vi "hamilton_controller_shunt2.vi"(8 "error in":errorcluster, 9 "Open?":bool, 10 "valve":enum16{"A", "B", "C", "D", "ALL", "E"}(ring), 11 "action":T1(ring)) -> (0 "error out":errorcluster)   [LabVIEW 2013]
uses:
  <vilib>/Instr/_visa.llb/VISA Configure Serial Port (Instr).vi
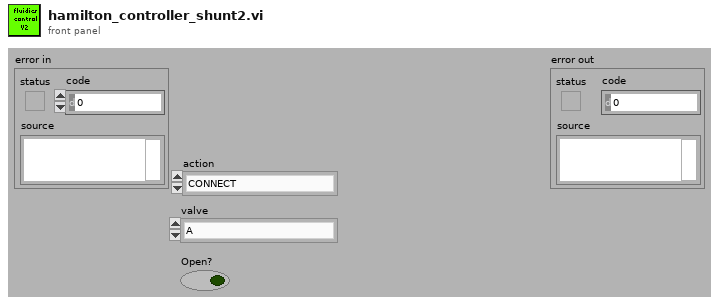
[diagram p1: front panel]
types:
  T1 = enum16{"CONNECT", "INITIALIZE VALVES", "DISCONNECT", "MOVE VALVE"}
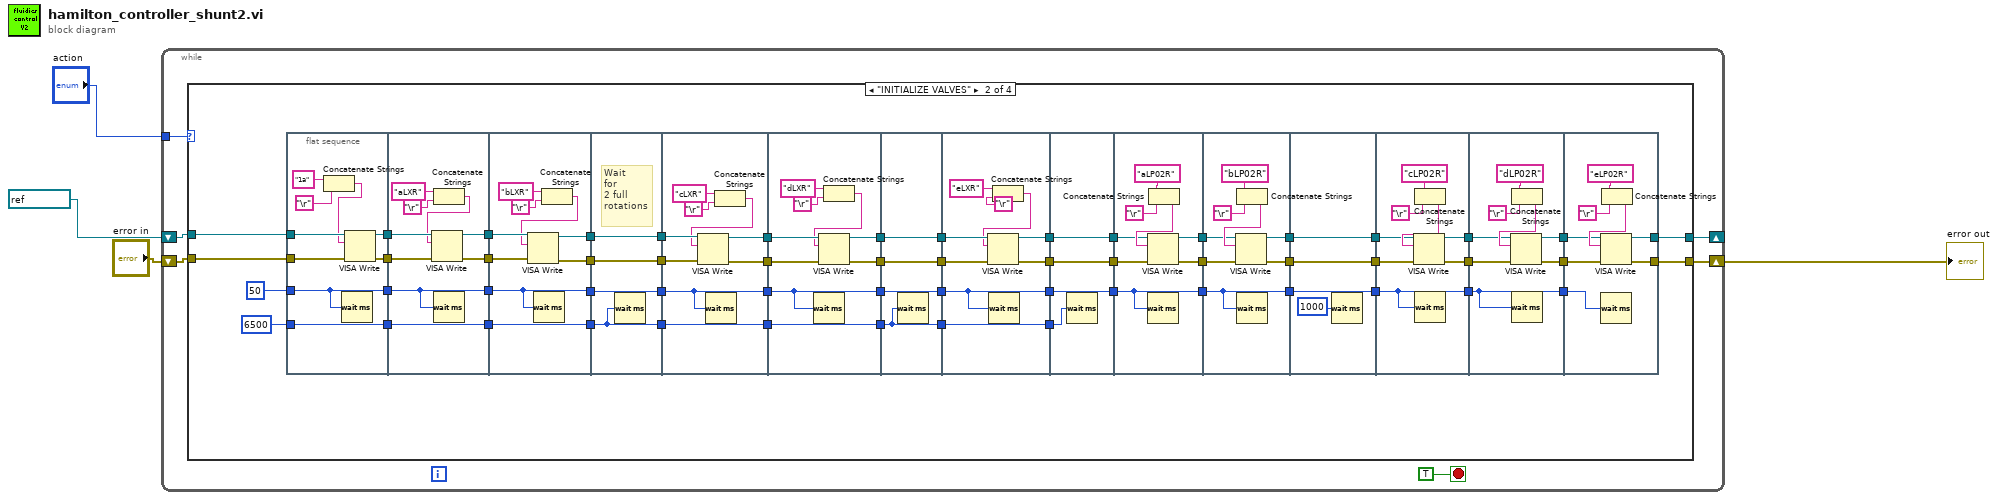
[diagram p0: block diagram]
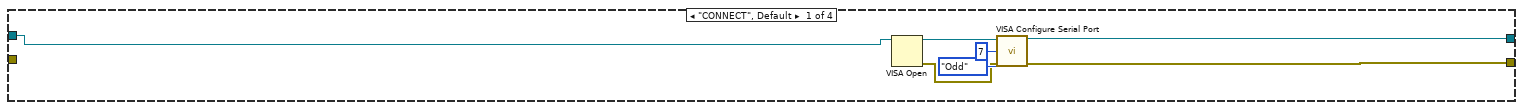
[diagram p2: hidden frame]
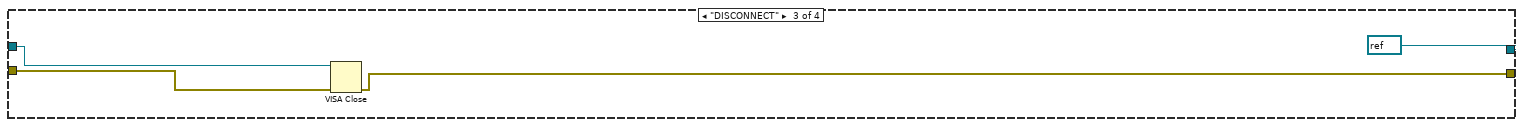
[diagram p3: hidden frame]
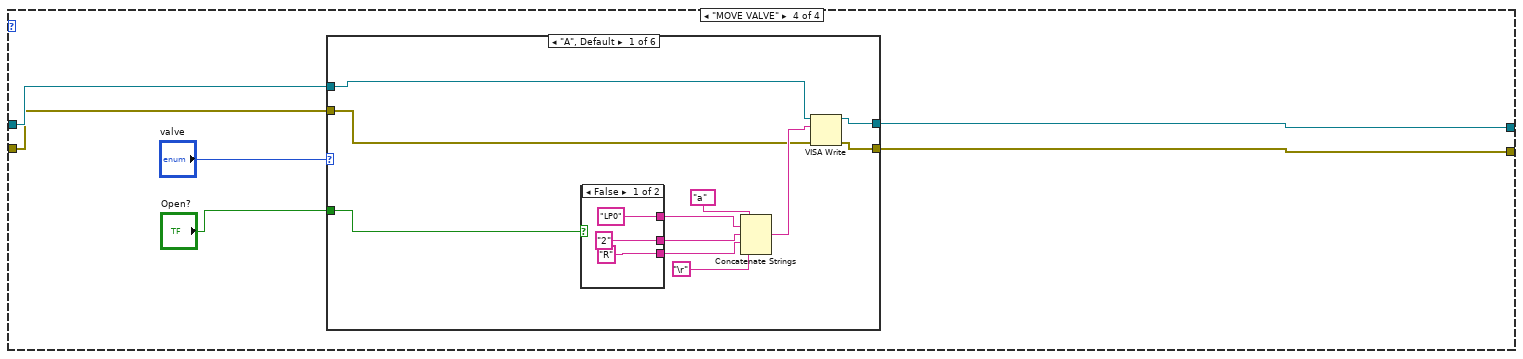
[diagram p4: hidden frame]
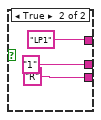
[diagram p5: hidden frame]
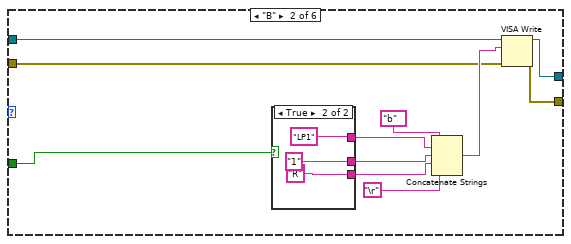
[diagram p6: hidden frame]
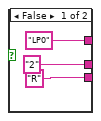
[diagram p7: hidden frame]
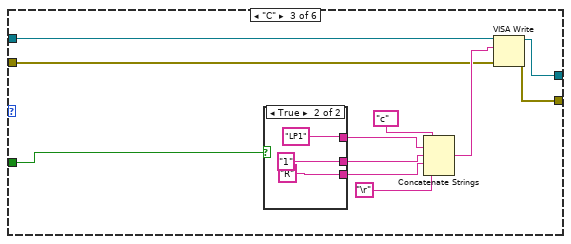
[diagram p8: hidden frame]
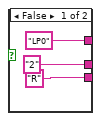
[diagram p9: hidden frame]
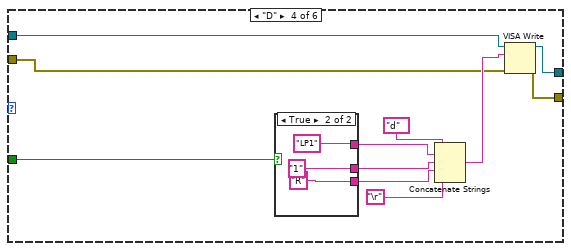
[diagram p10: hidden frame]
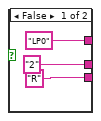
[diagram p11: hidden frame]
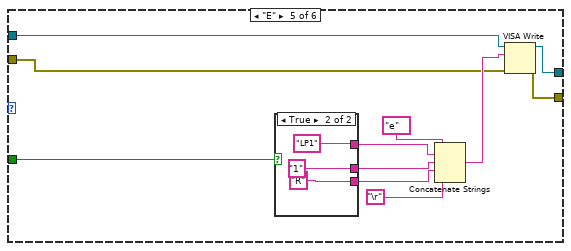
[diagram p12: hidden frame]
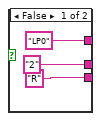
[diagram p13: hidden frame]
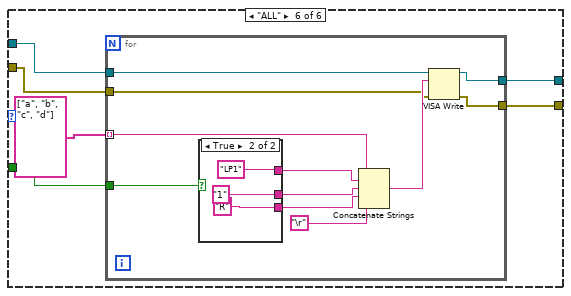
[diagram p14: hidden frame]
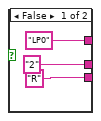
[diagram p15: hidden frame]
diagram:
  n1 = while {
    tunnel: "action" -> [w9]
    shift-right: [w8] -> _
    shift-left: refnum<visa-resource-name> "COM6" ("VISA resource name") -> [w6]
    shift-right: [w7] -> w2
    shift-left: "error in" -> [w5]
    stop <- TRUE stop-if-true
    n2 = case shown="\"INITIALIZE VALVES\"" w9 {
      tunnel: [w13 w46 refnum<visa-resource-name> refnum ("VISA resource name out") w190] -> w8
      tunnel: [w12 w45 w185 w189] -> w7
      tunnel: w6 -> [w11 w48 w187 w192]
      tunnel: w5 -> [_ w47 w186 w191]
      frame "CONNECT", Default {
        n3 = VISA Open(VISA resource name=w11) -> (VISA resource name=w17:refnum<visa-resource-name>, error out=w14:errorcluster)  [unwired: 4 in]
        n4 = call-poly "VISA Configure Serial Port"("VISA resource name"=w17, "data bits (8)"=u16 7, "parity (0:none)"=enum16{"None", "Odd", "Even", "Mark", "Space"}."Odd", "error in (no error)"=w14) -> ("VISA resource name out"=w13:refnum<visa-resource-name>, "error out"=w12:errorcluster)  [unwired: 10 in]
      }
      frame "INITIALIZE VALVES" {
        n5 = flat-sequence {
          tunnel: w48 -> [w82]
          tunnel: w47 -> [w81]
          tunnel: [w80] -> w73
          tunnel: [w76] -> w72
          tunnel: [w75] -> w33
          tunnel: u32 6500 ("milliseconds to wait") -> [w75]
          tunnel: u32 50 ("milliseconds to wait") -> [w74]
          tunnel: [w74] -> w26
          tunnel: w73 -> [w90]
          tunnel: w72 -> [w91]
          tunnel: [w83] -> w71
          tunnel: [w86] -> w70
          tunnel: [w85] -> w69
          tunnel: [w84] -> w34
          tunnel: w33 -> [w84]
          tunnel: w26 -> [w83]
          tunnel: w71 -> [w92]
          tunnel: w70 -> [w100]
          tunnel: [w99] -> w68
          tunnel: w69 -> [w98]
          tunnel: [w97] -> w67
          tunnel: [w92] -> w66
          tunnel: [w93] -> w35
          tunnel: w34 -> [w93]
          tunnel: w68 -> [w104]
          tunnel: [w104] -> w65
          tunnel: w67 -> [w103]
          tunnel: [w103] -> w64
          tunnel: w66 -> [w102]
          tunnel: [w102] -> w63
          tunnel: w35 -> [w101]
          tunnel: [w101] -> w25
          tunnel: w65 -> [w113]
          tunnel: [w112] -> w62
          tunnel: w64 -> [w111]
          tunnel: [w110] -> w61
          tunnel: w63 -> [w105]
          tunnel: [w106] -> w30
          tunnel: w25 -> [w106]
          tunnel: [w105] -> w24
          tunnel: w62 -> [w122]
          tunnel: w61 -> [w121]
          tunnel: [w117] -> w60
          tunnel: [w116] -> w59
          tunnel: [w115] -> w31
          tunnel: w30 -> [w115]
          tunnel: w24 -> [w114]
          tunnel: [w114] -> w23
          tunnel: w60 -> [w125]
          tunnel: w59 -> [w126]
          tunnel: [w126] -> w44
          tunnel: [w125] -> w43
          tunnel: w31 -> [w123]
          tunnel: [w124] -> w29
          tunnel: w23 -> [w124]
          tunnel: [w123] -> w22
          tunnel: w44 -> [w133]
          tunnel: [w130] -> w40
          tunnel: w43 -> [w132]
          tunnel: [w131] -> w37
          tunnel: w29 -> [w127]
          tunnel: [w128] -> w28
          tunnel: w22 -> [w128]
          tunnel: [w127] -> w21
          tunnel: w40 -> [w139]
          tunnel: [w139] -> w39
          tunnel: [w137] -> w38
          tunnel: w37 -> [w138]
          tunnel: [w138] -> w36
          tunnel: w28 -> [w136]
          tunnel: w21 -> [w137]
          tunnel: w39 -> [w143]
          tunnel: w38 -> [w140]
          tunnel: [w144] -> w58
          tunnel: [w140] -> w57
          tunnel: [w142] -> w56
          tunnel: w36 -> [w141]
          tunnel: w58 -> [w152]
          tunnel: w57 -> [w148]
          tunnel: [w151] -> w55
          tunnel: w56 -> [w150]
          tunnel: [w149] -> w54
          tunnel: [w148] -> w20
          tunnel: w55 -> [w159]
          tunnel: [w159] -> w53
          tunnel: [w158] -> w52
          tunnel: w54 -> [w157]
          tunnel: [w157] -> w51
          tunnel: w20 -> [w158]
          tunnel: w53 -> [w164]
          tunnel: w52 -> [w160]
          tunnel: [w163] -> w50
          tunnel: w51 -> [w162]
          tunnel: [w161] -> w49
          tunnel: [w160] -> w19
          tunnel: w50 -> [w172]
          tunnel: w49 -> [w170]
          tunnel: [w171] -> w42
          tunnel: [w169] -> w41
          tunnel: w19 -> [w168]
          tunnel: [w168] -> w18
          tunnel: [w179] -> w46
          tunnel: [w178] -> w45
          tunnel: w42 -> [w177]
          tunnel: w41 -> [w180]
          tunnel: w18 -> [w176]
          frame #0 {
            n6 = Concatenate Strings("1a" ("string"), "\r") -> (w77:string)
            n7 = Wait (ms)(milliseconds to wait=w74) -> ()  [unwired: 1 out]
            n8 = VISA Write(VISA resource name=w82, write buffer=w77, error in (no error)=w81) -> (VISA resource name out=w76:refnum<visa-resource-name>, error out=w80:errorcluster)  [unwired: 1 out]
          }
          frame #1 {
            n9 = Concatenate Strings("aLXR", "\r") -> (w87:string)
            n10 = VISA Write(VISA resource name=w91, write buffer=w87, error in (no error)=w90) -> (VISA resource name out=w86:refnum<visa-resource-name>, error out=w85:errorcluster)  [unwired: 1 out]
            n11 = Wait (ms)(milliseconds to wait=w83) -> ()  [unwired: 1 out]
          }
          frame #2 {
            n12 = Wait (ms)(milliseconds to wait=w92) -> ()  [unwired: 1 out]
            n13 = Concatenate Strings("bLXR", "\r") -> (w94:string)
            n14 = VISA Write(VISA resource name=w100, write buffer=w94, error in (no error)=w98) -> (VISA resource name out=w99:refnum<visa-resource-name>, error out=w97:errorcluster)  [unwired: 1 out]
          }
          frame #3 {
            # "Wait\nfor\n2 full\nrotations"
            n15 = Wait (ms)(milliseconds to wait=w101) -> ()  [unwired: 1 out]
          }
          frame #4 {
            n16 = Wait (ms)(milliseconds to wait=w105) -> ()  [unwired: 1 out]
            n17 = Concatenate Strings("cLXR", "\r") -> (w107:string)
            n18 = VISA Write(VISA resource name=w113, write buffer=w107, error in (no error)=w111) -> (VISA resource name out=w112:refnum<visa-resource-name>, error out=w110:errorcluster)  [unwired: 1 out]
          }
          frame #5 {
            n19 = Wait (ms)(milliseconds to wait=w114) -> ()  [unwired: 1 out]
            n20 = Concatenate Strings("dLXR", "\r") -> (w118:string)
            n21 = VISA Write(VISA resource name=w122, write buffer=w118, error in (no error)=w121) -> (VISA resource name out=w116:refnum<visa-resource-name>, error out=w117:errorcluster)  [unwired: 1 out]
          }
          frame #6 {
            n22 = Wait (ms)(milliseconds to wait=w123) -> ()  [unwired: 1 out]
          }
          frame #7 {
            n23 = Wait (ms)(milliseconds to wait=w127) -> ()  [unwired: 1 out]
            n24 = Concatenate Strings("eLXR", "\r") -> (w129:string)
            n25 = VISA Write(VISA resource name=w133, write buffer=w129, error in (no error)=w132) -> (VISA resource name out=w130:refnum<visa-resource-name>, error out=w131:errorcluster)  [unwired: 1 out]
          }
          frame #8 {
            n26 = Wait (ms)(milliseconds to wait=w136) -> ()  [unwired: 1 out]
          }
          frame #9 {
            n27 = Wait (ms)(milliseconds to wait=w140) -> ()  [unwired: 1 out]
            n28 = Concatenate Strings("aLP02R" ("string"), "\r") -> (w147:string)
            n29 = VISA Write(VISA resource name=w143, write buffer=w147, error in (no error)=w141) -> (VISA resource name out=w142:refnum<visa-resource-name>, error out=w144:errorcluster)  [unwired: 1 out]
          }
          frame #10 {
            n30 = Concatenate Strings("bLP02R" ("string"), "\r") -> (w155:string)
            n31 = VISA Write(VISA resource name=w150, write buffer=w155, error in (no error)=w152) -> (VISA resource name out=w149:refnum<visa-resource-name>, error out=w151:errorcluster)  [unwired: 1 out]
            n32 = Wait (ms)(milliseconds to wait=w148) -> ()  [unwired: 1 out]
          }
          frame #11 {
            n33 = Wait (ms)(milliseconds to wait=u32 1000) -> ()  [unwired: 1 out]
          }
          frame #12 {
            n34 = Concatenate Strings("cLP02R" ("string"), "\r") -> (w167:string)
            n35 = VISA Write(VISA resource name=w162, write buffer=w167, error in (no error)=w164) -> (VISA resource name out=w161:refnum<visa-resource-name>, error out=w163:errorcluster)  [unwired: 1 out]
            n36 = Wait (ms)(milliseconds to wait=w160) -> ()  [unwired: 1 out]
          }
          frame #13 {
            n37 = Concatenate Strings("dLP02R" ("string"), "\r") -> (w175:string)
            n38 = VISA Write(VISA resource name=w170, write buffer=w175, error in (no error)=w172) -> (VISA resource name out=w169:refnum<visa-resource-name>, error out=w171:errorcluster)  [unwired: 1 out]
            n39 = Wait (ms)(milliseconds to wait=w168) -> ()  [unwired: 1 out]
          }
          frame #14 {
            n40 = Wait (ms)(milliseconds to wait=w176) -> ()  [unwired: 1 out]
            n41 = Concatenate Strings("eLP02R" ("string"), "\r") -> (w181:string)
            n42 = VISA Write(VISA resource name=w180, write buffer=w181, error in (no error)=w177) -> (VISA resource name out=w179:refnum<visa-resource-name>, error out=w178:errorcluster)  [unwired: 1 out]
          }
        }
      }
      frame "DISCONNECT" {
        n43 = VISA Close(VISA resource name=w187, error in (no error)=w186) -> (error out=w185:errorcluster)
      }
      frame "MOVE VALVE" {
        n44 = case shown="\"A\", Default" "valve" {
          tunnel: w192 -> [w198 w215 w230 w249 w266 w284]
          tunnel: w191 -> [w197 w214 w229 w248 w265 w281]
          tunnel: [w196 w213 w232 w247 w264 w279] -> w190
          tunnel: [w195 w212 w231 w246 w263 w280] -> w189
          tunnel: "Open?" -> [w194 w211 w228 w245 w262 w283]
          frame "A", Default {
            n45 = case shown="False" w194 {
              tunnel: ["R" "R"] -> w202
              tunnel: ["2" "1"] -> w203
              tunnel: ["LP0" ("string") "LP1" ("string")] -> w200
              frame False {
              }
              frame True {
              }
            }
            n46 = Concatenate Strings("a" ("MVP ID"), w200, w203, w202, "\r") -> (w199:string)
            n47 = VISA Write(VISA resource name=w198, write buffer=w199, error in (no error)=w197) -> (VISA resource name out=w196:refnum<visa-resource-name>, error out=w195:errorcluster)  [unwired: 1 out]
          }
          frame "B" {
            n48 = case shown="True" w211 {
              tunnel: ["R" "R"] -> w219
              tunnel: ["2" "1"] -> w220
              tunnel: ["LP0" ("string") "LP1" ("string")] -> w217
              frame False {
              }
              frame True {
              }
            }
            n49 = Concatenate Strings("b" ("MVP ID"), w217, w220, w219, "\r") -> (w216:string)
            n50 = VISA Write(VISA resource name=w215, write buffer=w216, error in (no error)=w214) -> (VISA resource name out=w213:refnum<visa-resource-name>, error out=w212:errorcluster)  [unwired: 1 out]
          }
          frame "C" {
            n51 = case shown="True" w228 {
              tunnel: ["R" "R"] -> w236
              tunnel: ["2" "1"] -> w237
              tunnel: ["LP0" ("string") "LP1" ("string")] -> w234
              frame False {
              }
              frame True {
              }
            }
            n52 = Concatenate Strings("c" ("MVP ID"), w234, w237, w236, "\r") -> (w233:string)
            n53 = VISA Write(VISA resource name=w230, write buffer=w233, error in (no error)=w229) -> (VISA resource name out=w232:refnum<visa-resource-name>, error out=w231:errorcluster)  [unwired: 1 out]
          }
          frame "D" {
            n54 = case shown="True" w245 {
              tunnel: ["R" "R"] -> w253
              tunnel: ["2" "1"] -> w254
              tunnel: ["LP0" ("string") "LP1" ("string")] -> w251
              frame False {
              }
              frame True {
              }
            }
            n55 = Concatenate Strings("d" ("MVP ID"), w251, w254, w253, "\r") -> (w250:string)
            n56 = VISA Write(VISA resource name=w249, write buffer=w250, error in (no error)=w248) -> (VISA resource name out=w247:refnum<visa-resource-name>, error out=w246:errorcluster)  [unwired: 1 out]
          }
          frame "E" {
            n57 = case shown="True" w262 {
              tunnel: ["R" "R"] -> w270
              tunnel: ["2" "1"] -> w271
              tunnel: ["LP0" ("string") "LP1" ("string")] -> w268
              frame False {
              }
              frame True {
              }
            }
            n58 = Concatenate Strings("e" ("MVP ID"), w268, w271, w270, "\r") -> (w267:string)
            n59 = VISA Write(VISA resource name=w266, write buffer=w267, error in (no error)=w265) -> (VISA resource name out=w264:refnum<visa-resource-name>, error out=w263:errorcluster)  [unwired: 1 out]
          }
          frame "ALL" {
            n60 = for {
              tunnel: w284 -> [w291]
              tunnel: w283 -> [w290]
              tunnel: string[] ["a", "b", "c", "d"] -> [w289] mode=indexing
              tunnel: w281 -> [w287]
              tunnel: [w286] -> w280
              tunnel: [w285] -> w279
              n61 = case shown="True" w290 {
                tunnel: ["R" "R"] -> w294
                tunnel: ["2" "1"] -> w295
                tunnel: ["LP0" ("string") "LP1" ("string")] -> w292
                frame False {
                }
                frame True {
                }
              }
              n62 = Concatenate Strings(w289, w292, w295, w294, "\r") -> (w288:string)
              n63 = VISA Write(VISA resource name=w291, write buffer=w288, error in (no error)=w287) -> (VISA resource name out=w285:refnum<visa-resource-name>, error out=w286:errorcluster)  [unwired: 1 out]
            }
          }
        }
      }
    }
  }
  "error out" <- w2
